vi "SaveDataHD.vi"(10 "Array":T2(array[cluster]), 11 "Type of scan":T1=enum."M scan") -> (3 "Aborted":bool)   [LabVIEW 2022 SP3]
uses:
  Controls/ScanType2.ctl
  Motion Controllers/-MotionRoutines/MotionGlobals.vi
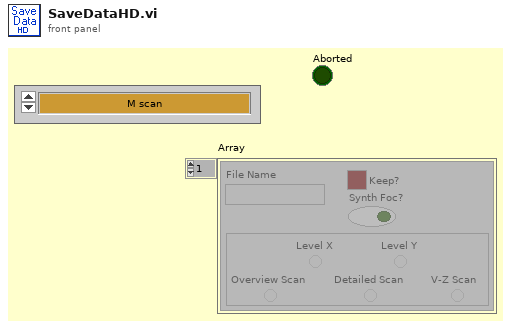
[diagram p1: front panel]
types:
  T1 = typedef "ScanType2.ctl" = enum16{"Therapy With Scan", "M scan", "M Scan With Therapy Burst", "1-D B Scan", "1-D B Scan With Therapy Burst", "2-D B Scan", "2-D B Scan With Therapy Burst", "Rotational Scan", "1-D B-Scan PRF", "2-D B-Scan PRF", "Real-Time Scan", "Contrast Agents", "1-D w/ Real-Time Set Up", "Dual Transducer", "Acoustic Microscopy", "Hydrophone Scanning"}
  T2 = cluster{"File Name":string, "Keep?":bool, "Synth Foc?":bool, "Microscopy Scan Mode":enum32{"Level X", "Level Y", "Overview Scan", "Detailed Scan", "V-Z Scan"}}[]
  T3 = typedef "location.ctl" = enum16{"Automatic", "WCM Main", "Hawaii", "Columbia MM3000", "Columbia  NI System", "NYU", "RRI 2", "UHI Allen", "CUMC RT", "Chiba", "Stony Brook", "WCM Microscopy", "WCM Aeoretch", "WCM Optics Lab", "WCM Main 2Axis", "WCM Rotation", "WCM SAM SMAC", "SERI GP"}
  T4 = enum32{"Level X", "Level Y", "Overview Scan", "Detailed Scan", "V-Z Scan"}
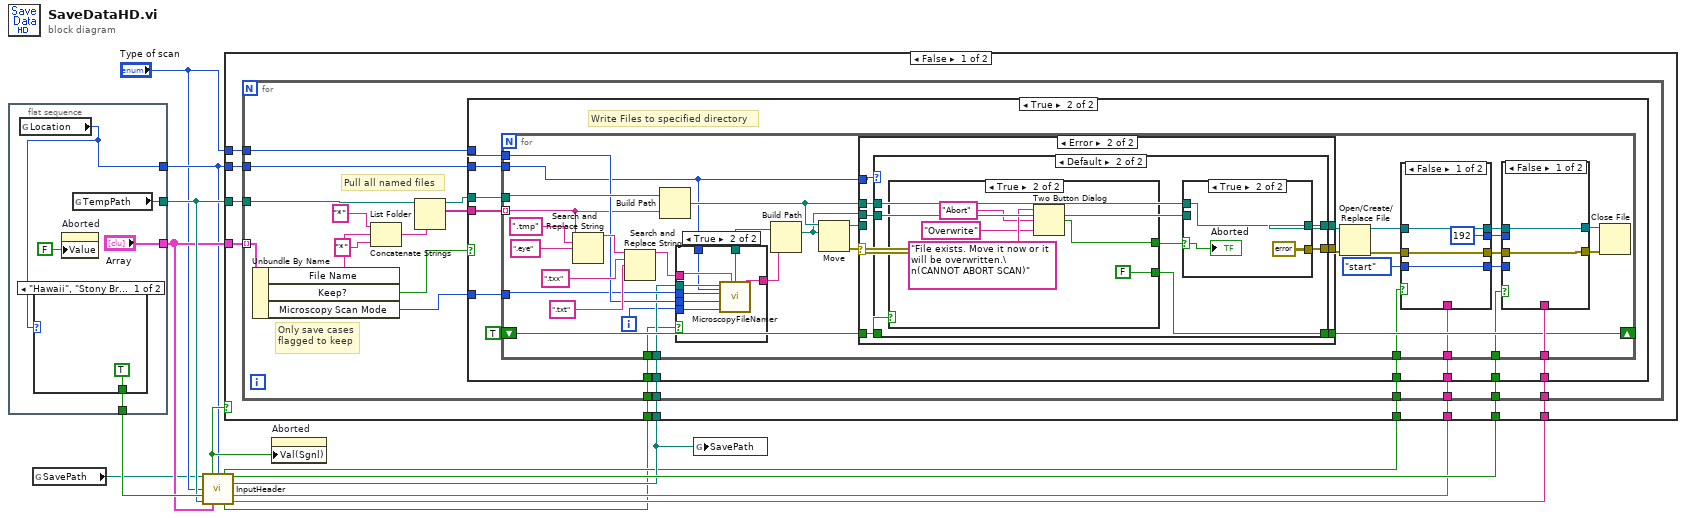
[diagram p0: block diagram]
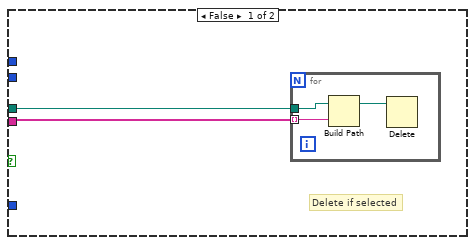
[diagram p2: hidden frame]
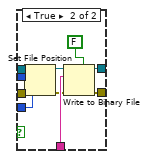
[diagram p4: hidden frame]
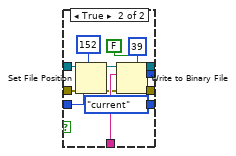
[diagram p5: hidden frame]
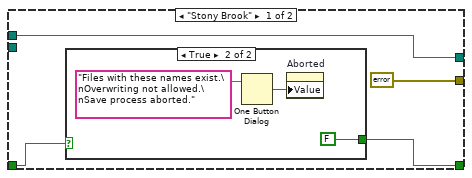
[diagram p7: hidden frame]
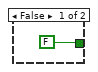
[diagram p8: hidden frame]
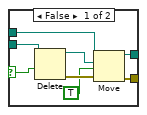
[diagram p9: hidden frame]
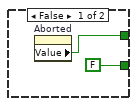
[diagram p10: hidden frame]
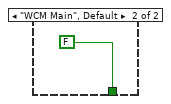
[diagram p12: hidden frame]
diagram:
  n1 = flat-sequence {
    tunnel: ["Array"] -> w4
    tunnel: [w17] -> w5
    tunnel: [w15] -> w3
    tunnel: [w14] -> w11
    frame #0 {
      n2 = global read "MotionGlobals.vi" "Location"() -> (w15:T3)
      n3 = case shown="\"Hawaii\", \"Stony Brook\"" w15 {
        tunnel: [TRUE FALSE] -> w14
        frame "Hawaii", "Stony Brook" {
        }
        frame "WCM Main", Default {
        }
      }
      n4 = property on="Aborted" class="Bool (strict)"("Value"=FALSE ("Aborted")) -> ()  [unwired: 2 in, 2 out]
      n5 = global read "MotionGlobals.vi" "TempPath"() -> (w17:path)
    }
  }
  n6 = global read "MotionGlobals.vi" "SavePath"() -> (w1:path)
  n7 = call "InputHeader.vi"("Save Path"=w1, "Location"=w3, "Type of scan"="Type of scan", "LOS Visable?"=w11, "TempPath"=w5, "Array"=w4) -> ("Aborted?"=w10:bool, "Write LOS?"=w7:bool, "Write Comment?"=w13:bool, "Save Path Out"=w12:path, "LOS"=w9:string, "Use Dual Mode Folders?"=w6:bool, "Comment out"=w8:string)  [unwired: 3 in]
  n8 = case shown="False" w10 {
    tunnel: w4 -> [w30 _]
    tunnel: w13 -> [w29 _]
    tunnel: w8 -> [w28 _]
    tunnel: w5 -> [w27 _]
    tunnel: w12 -> [w26 _]
    tunnel: w3 -> [w25 _]
    tunnel: w9 -> [w24 _]
    tunnel: w7 -> [w23 _]
    tunnel: w6 -> [w22 _]
    tunnel: "Type of scan" -> [w21 _]
    frame False {
      n9 = for {
        tunnel: w30 -> [w48] mode=indexing
        tunnel: w26 -> [w37]
        tunnel: w28 -> [w46]
        tunnel: w29 -> [w45]
        tunnel: w27 -> [w43]
        tunnel: w25 -> [w36]
        tunnel: w24 -> [w35]
        tunnel: w23 -> [w34]
        tunnel: w22 -> [w33]
        tunnel: w21 -> [w32]
        # "Pull all named files"
        # "Only save cases\nflagged to keep"
        n10 = Unbundle By Name(w48) -> ("File Name"=w40:string, "Keep?"=w47:bool, "Microscopy Scan Mode"=w31:T4)
        n11 = Concatenate Strings("*", w40, "*") -> (w42:string)
        n12 = List Folder(path=w43, pattern=w42) -> (path out=w39:path, filenames=w41:string[])  [unwired: 1 in, 3 out]
        n13 = case shown="True" w47 {
          tunnel: w37 -> [_ w65]
          tunnel: w46 -> [_ w64]
          tunnel: w45 -> [_ w63]
          tunnel: w39 -> [w50 w62]
          tunnel: w41 -> [w49 w61]
          tunnel: w36 -> [_ w59]
          tunnel: w31 -> [_ w58]
          tunnel: w32 -> [_ w57]
          tunnel: w35 -> [_ w56]
          tunnel: w34 -> [_ w55]
          tunnel: w33 -> [_ w54]
          frame False {
            # "Delete if selected"
            n14 = for {
              tunnel: w50 -> [w53]
              tunnel: w49 -> [w52] mode=indexing
              n15 = Build Path(base path=w53, name or relative path=w52) -> (appended path=w51:path)
              n16 = Delete(path (use dialog)=w51) -> ()  [unwired: 1 in, 6 out]
            }
          }
          frame True {
            # "Write Files to specified directory"
            n17 = for {
              tunnel: w65 -> [w86]
              tunnel: w64 -> [w99]
              tunnel: w63 -> [w69]
              tunnel: w61 -> [w82] mode=indexing
              tunnel: w62 -> [w95]
              shift-right: [w89] -> _
              shift-left: TRUE -> [w90]
              tunnel: w59 -> [w68]
              tunnel: w58 -> [w87]
              tunnel: w57 -> [w88]
              tunnel: w56 -> [w80]
              tunnel: w55 -> [w70]
              tunnel: w54 -> [w67]
              i -> [w84]
              n18 = Search and Replace String(input string=w82, search string=".tmp", replace string=".eye") -> (result string=w93:string)  [unwired: 1 in, 7 out]
              n19 = Search and Replace String(input string=w93, search string=".txx", replace string=".txt") -> (result string=w81:string)  [unwired: 1 in, 7 out]
              n20 = Build Path(base path=w95, name or relative path=w82) -> (appended path=w96:path)
              n21 = case shown="True" w67 {
                tunnel: w88 -> [_ w112]
                tunnel: w87 -> [_ w111]
                tunnel: w86 -> [w104 w110]
                tunnel: [w104 w109] -> w85
                tunnel: w84 -> [_ w108]
                tunnel: [w103 w107] -> w83
                tunnel: w81 -> [w103 w106]
                tunnel: w68 -> [_ w105]
                frame False {
                }
                frame True {
                  n22 = call "MicroscopyFileNamer.vi"("Location"=w105, "String in"=w106, "FileCount"=w108, "Type of scan"=w112, "Microscopy Scan Mode"=w111, "Save Path In"=w110) -> ("FIle Name out"=w107:string, "Scan Data Path"=w109:path)  [unwired: 4 in]
                }
              }
              n23 = Build Path(base path=w85, name or relative path=w83) -> (appended path=w66:path)
              n24 = Move(source path=w96, 10:w66) -> (error out=w102:errorcluster, 3:w101:path)  [unwired: 1 in, 3 out]
              n25 = case shown="Error" w102 {
                selector: w102 -> [w142 _]
                tunnel: w101 -> [w143 _]
                tunnel: [w143 w149] -> w100
                tunnel: w96 -> [_ w150]
                tunnel: w66 -> [_ w148]
                tunnel: [w142 w147] -> w91
                tunnel: w90 -> [w141 w146]
                tunnel: [w141 w145] -> w89
                tunnel: w68 -> [_ w144]
                frame No Error {
                }
                frame Error {
                  n26 = case shown="Default" w144 {
                    tunnel: w150 -> [w154 w165]
                    tunnel: [w154 w164] -> w149
                    tunnel: w148 -> [_ w163]
                    tunnel: [errorcluster {"status"=FALSE, "code"=0, "source"=""} ("error out") w162] -> w147
                    tunnel: w146 -> [w152 w161]
                    tunnel: [w151 w160] -> w145
                    frame "Stony Brook" {
                      n27 = case shown="True" w152 {
                        tunnel: [FALSE FALSE] -> w151
                        frame False {
                        }
                        frame True {
                          n28 = One Button Dialog(message="Files with these names exist.\nOverwriting not allowed.\nSave process aborted.") -> (true=w156:bool)  [unwired: 1 in]
                          n29 = property on="Aborted" class="Bool (strict)"("Value"=w156) -> ()  [unwired: 2 in, 2 out]
                        }
                      }
                    }
                    frame Default {
                      n30 = case shown="True" w161 {
                        tunnel: [w177 w179] -> w159
                        tunnel: [FALSE FALSE] -> w160
                        frame False {
                          n31 = property on="Aborted" class="Bool (strict)"() -> ("Value"=w177:bool)  [unwired: 2 in, 2 out]
                        }
                        frame True {
                          n32 = Two Button Dialog(message="File exists. Move it now or it will be overwritten.\n(CANNOT ABORT SCAN)", 1:"Overwrite" ("T button name (\"OK\")"), 2:"Abort" ("F button name (\"Cancel\")")) -> (T button?=w179:bool)
                        }
                      }
                      n33 = case shown="True" w159 {
                        selector: w159 -> [w166 w174]
                        tunnel: w165 -> [w173 w176]
                        tunnel: [w172 w176] -> w164
                        tunnel: w163 -> [w171 _]
                        tunnel: [w170 errorcluster {"status"=FALSE, "code"=0, "source"=""} ("error out")] -> w162
                        frame False {
                          n34 = Delete(path (use dialog)=w171, confirm (F)=w166) -> (deleted path=w168:path, error out=w169:errorcluster)  [unwired: 2 in, 2 out]
                          n35 = Move(source path=w173, error in=w169, 9:TRUE, 10:w168) -> (error out=w170:errorcluster, 3:w172:path)  [unwired: 2 out]
                        }
                        frame True {
                          "Aborted" <- w174
                        }
                      }
                    }
                  }
                }
              }
              n36 = Open/Create/Replace File(file path (use dialog)=w100, error in=w91) -> (refnum out=w77:refnum<file>, error out=w76:errorcluster)  [unwired: 5 out]
              n37 = case shown="False" w70 {
                tunnel: w80 -> [_ w140]
                tunnel: [192 39] -> w79
                tunnel: [w126 w134] -> w78
                tunnel: w77 -> [w126 w133]
                tunnel: w76 -> [w127 w132]
                tunnel: [w127 w131] -> w75
                tunnel: [w128 enum16{"start", "end", "current"}."current" ("from (0:start)")] -> w74
                tunnel: enum16{"start", "end", "current"}."start" ("from (0:start)") -> [w128 w129]
                frame False {
                }
                frame True {
                  n38 = Set File Position(offset (in bytes) (0)=152, refnum=w133, from (0:start)=w129, error in=w132) -> (refnum out=w138:refnum<file>, error out=w137:errorcluster)
                  n39 = Write to Binary File(file (use dialog)=w138, data=w140, error in=w137, 5:FALSE ("prepend array or string size? (T)")) -> (refnum out=w134:refnum<file>, error out=w131:errorcluster)  [unwired: 3 out]
                }
              }
              n40 = case shown="False" w69 {
                tunnel: w99 -> [_ w124]
                tunnel: w79 -> [_ w123]
                tunnel: w78 -> [w114 w122]
                tunnel: w75 -> [w113 w121]
                tunnel: w74 -> [_ w120]
                tunnel: [w114 w119] -> w72
                tunnel: [w113 w118] -> w71
                frame False {
                }
                frame True {
                  n41 = Set File Position(offset (in bytes) (0)=w123, refnum=w122, from (0:start)=w120, error in=w121) -> (refnum out=w117:refnum<file>, error out=w116:errorcluster)
                  n42 = Write to Binary File(file (use dialog)=w117, data=w124, error in=w116, 5:FALSE ("prepend array or string size? (T)")) -> (refnum out=w119:refnum<file>, error out=w118:errorcluster)  [unwired: 3 out]
                }
              }
              n43 = Close File(refnum=w72, error in=w71) -> ()  [unwired: 2 out]
            }
          }
        }
      }
    }
    frame True {
    }
  }
  n44 = property on="Aborted" class="Bool (strict)"("Val(Sgnl)"=w10) -> ()  [unwired: 2 in, 2 out]
  n45 = global write "MotionGlobals.vi" "SavePath"(w12) -> ()
